vi "Draw.vi"(8 "error in (no error)":errorcluster, 11 "Circle in":refnum<class "Circle.lvclass">) -> (0 "error out":errorcluster, 2 "Picture":picture, 3 "Circle out":refnum<class "Circle.lvclass">)   [LabVIEW 2015, in "Circle.lvclass"]
uses:
  Circle.lvclass
  <vilib>/LIEF/Forms/Shape/Shape.lvclass/Shape.ctl
  Circle.lvclass/Circle.ctl
  <vilib>/LIEF/Forms/Shape/Read Color.vi
  <vilib>/LIEF/Forms/Layered Shape/Layered Shape.lvclass
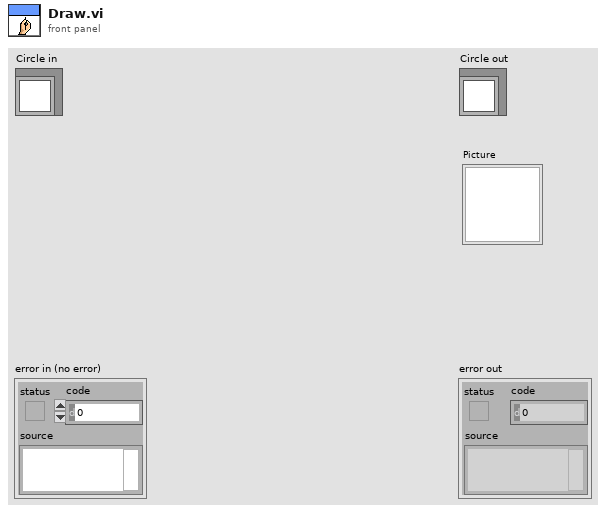
[diagram p1: front panel]
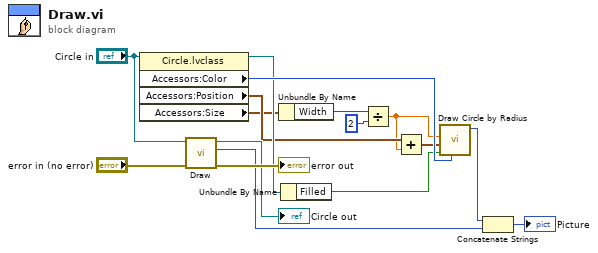
[diagram p0: block diagram]
diagram:
  n1 = property class="Circle.lvclass"(reference="Circle in") -> (reference out=w8:refnum<class "Circle.lvclass">, "Accessors:Color"=w9:u32, "Accessors:Position"=w6:cluster{"Left":i32, "Top":i32}, "Accessors:Size"=w4:cluster{"Width":i32, "Height":i32})  [unwired: 1 in, 1 out]
  n2 = call-parent "Draw.vi"("error in (no error)"="error in (no error)", "Layered Shape in"="Circle in") -> ("error out"=→"error out":errorcluster, "Picture"=w10:picture, "Layered Shape out"=→"Circle out":refnum<class "Circle.lvclass">)  [unwired: 7 in]
  n3 = Unbundle By Name(w4) -> ("Width"=w2:i32)
  n4 = Unbundle By Name(w8) -> ("Filled"=w7:bool)
  n5 = Divide(x=w2, y=2) -> (x/y=w1:dbl)
  n6 = Add(x=w6, y=w1) -> (x+y=w5:cluster{"Left":dbl, "Top":dbl})
  n7 = call <vilib>:"Draw Circle by Radius.vi"("color(black)"=w9, "fill?(F)"=w7, "pixel center"=w5, "radius"=w1) -> ("new picture"=w12:picture)  [unwired: 7 in]
  n8 = Concatenate Strings(w12, w10) -> (→"Picture":picture)
